vi "DN4_ControlStart.vi"(2 "error in (no error)":errorcluster, 4 "Task ID":u32) -> (0 "error out":errorcluster, 1 "Task ID":u32)   [LabVIEW 2009]
uses:
  Windows/System32/AdvLvDaq.dll
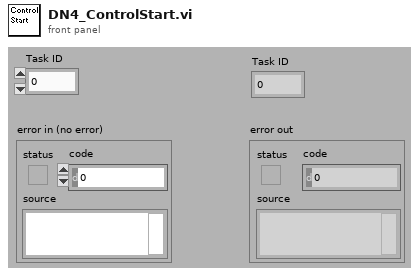
[diagram p1: front panel]
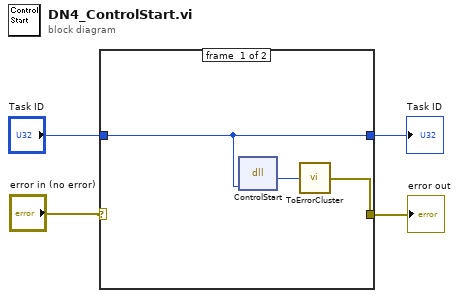
[diagram p0: block diagram]
diagram:
  n1 = case shown="No Error" "error in (no error)" {
    selector: "error in (no error)" -> [_ w8]
    tunnel: "Task ID" -> [w7 w9]
    tunnel: [w7 w9] -> w2
    tunnel: [w5 w8] -> w1
    frame #0 {
      n2 = dll-call lib="C:/Windows/System32/AdvLvDaq.dll" fn="ControlStart"("taskId"=w7) -> ("return type"=w6:i32)  [unwired: 4 in, 2 out]
      n3 = call <userlib>:"ToErrorCluster.vi"("error code"=w6) -> ("error out"=w5:errorcluster)
    }
    frame #1 {
    }
  }
  "error out" <- w1
  "Task ID" <- w2
